vi "GetSensorTrendNames.vi"(7 "service":refnum<class "IcmMessageService.lvclass">, 8 "error in (no error)":errorcluster, 10 "equip id":string, 11 "sensor names in":variant) -> (0 "error out":errorcluster, 2 "trend names":variant, 3 "sensor names out":variant)   [LabVIEW 2016]
doc: "Gets and caches the feature names for a specific equipment asset node."
uses:
  <vilib>/addons/InsightCM/MessageBus/MessageService/IcmMessageService.lvclass
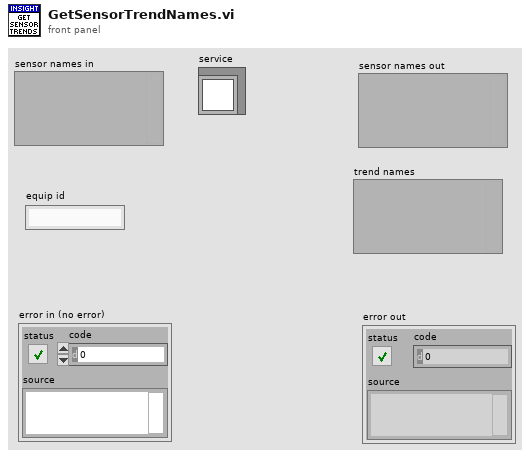
[diagram p1: front panel]
types:
  T1 = typedef "AssetNodeView.ctl" = cluster{"Id":string, "Type":string, "Name":string, "ParentIds":string[], "State":T2, "MeasType":string, "Metrics":T3[], "References":T5[], "HasOperatingStates":bool}
  T2 = typedef "AssetState.ctl" = cluster{"Disabled":bool}
  T3 = typedef "Metric.ctl" = cluster{"Id":string, "Name":string, "Unit":string, "Properties":T4[], "MetricDefinitionInstanceId":string}
  T4 = typedef "KeyValuePair.ctl" = cluster{"Key":string, "Value":string}
  T5 = typedef "AssetNodeReference.ctl" = cluster{"NodeId":string, "Name":string}
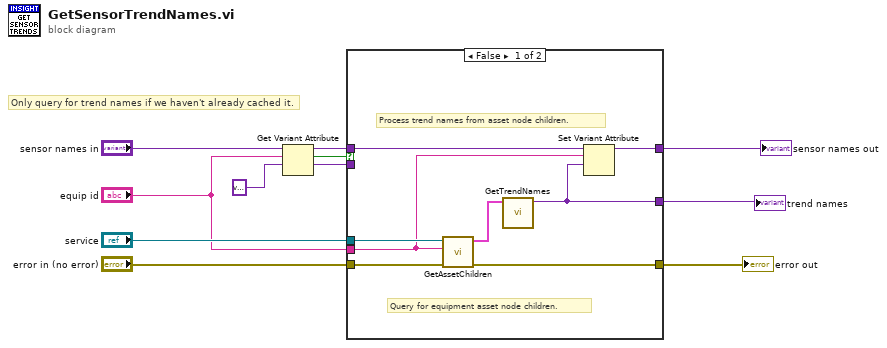
[diagram p0: block diagram]
diagram:
  # "Only query for trend names if we haven't already cached it."
  n1 = Get Variant Attribute(Variant="sensor names in", name="equip id", default value (empty Variant)=variant ("sensor names in")) -> (duplicate Variant=w5:variant, found=w9:bool, value=w2:variant)  [unwired: 1 in, 1 out]
  n2 = case shown="False" w9 {
    tunnel: "service" -> [w19 _]
    tunnel: "equip id" -> [w15 _]
    tunnel: "error in (no error)" -> [w18 w20]
    tunnel: w5 -> [w16 w22]
    tunnel: [w14 w22] -> w4
    tunnel: [w13 w21] -> w3
    tunnel: w2 -> [_ w21]
    tunnel: [w12 w20] -> w1
    frame False {
      # "Process trend names from asset node children."
      # "Query for equipment asset node children."
      n3 = call "GetAssetChildren.vi"("error in (no error)"=w18, "parent id"=w15, "service"=w19) -> ("error out"=w12:errorcluster, "AssetNodes"=w17:T1[])  [unwired: 7 in]
      n4 = call "GetTrendNames.vi"("AssetNodes"=w17) -> ("trend names"=w13:variant)  [unwired: 10 in]
      n5 = Set Variant Attribute(Variant=w16, name=w15, value=w13) -> (Variant out=w14:variant)  [unwired: 1 in, 2 out]
    }
    frame True {
    }
  }
  "sensor names out" <- w4
  "trend names" <- w3
  "error out" <- w1
